vi "ACP Configure.vi"(0 "RFmx Handle In":refnum<k21>, 1 "Selector String":string, 5 "RFmx LTE ACP Configuration":T1={"Measurement Enabled"=TRUE, "Number of GSM Offsets"=0, "Number of UTRA Offsets"=2, "Number of EUTRA Offsets"=1, "Sweep Time Auto"=1, "Sweep Time Interval (s)"=0.001, "Averaging Enabled"=0, "Averaging Count"=10, "Averaging Type"=0, "RBW Auto"=1, "RBW (Hz)"=30000.0, "RBW Filter Type"=0} {"RBW Filter Type" items=["FFT Based", "Gaussian", "Flat"]; "RBW Auto" items=["False", "True"]; "Averaging Type" items=["False", "True"]; "Averaging Enabled" items=["False", "True"]; "Sweep Time Auto" items=["False", "True"]}, 11 "error in (no error)":errorcluster) -> (4 "RFmx Handle Out":refnum<k21>, 15 "error out":errorcluster)   [LabVIEW 2018, in "RFmxLTE.lvlib"]
uses:
  RFmxLTE.lvlib
  Typedefs/ACP Configuration.ctl
  <resource>/objmgr/RFmxLTE.rc
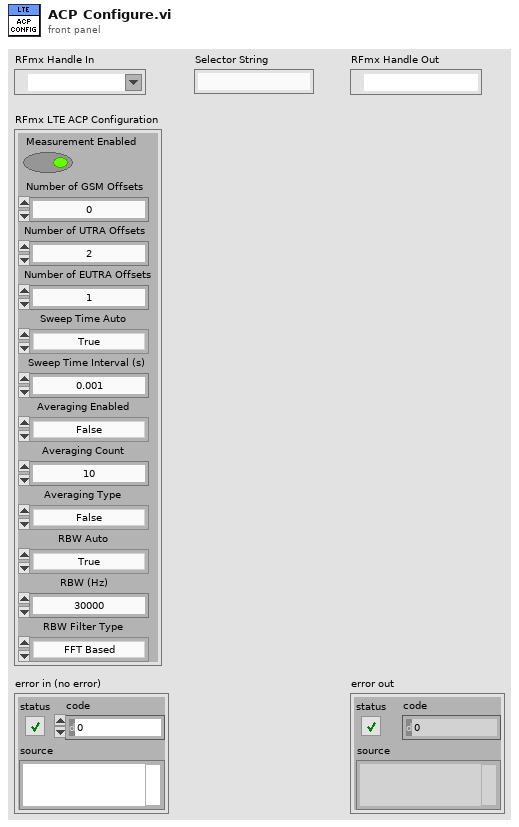
[diagram p1: front panel]
types:
  T1 = typedef "RFmxLTE.lvlib/ACP Configuration.ctl" = cluster{"Measurement Enabled":bool, "Number of GSM Offsets":i32, "Number of UTRA Offsets":i32, "Number of EUTRA Offsets":i32, "Sweep Time Auto":i32, "Sweep Time Interval (s)":dbl, "Averaging Enabled":i32, "Averaging Count":i32, "Averaging Type":i32, "RBW Auto":i32, "RBW (Hz)":dbl, "RBW Filter Type":i32}
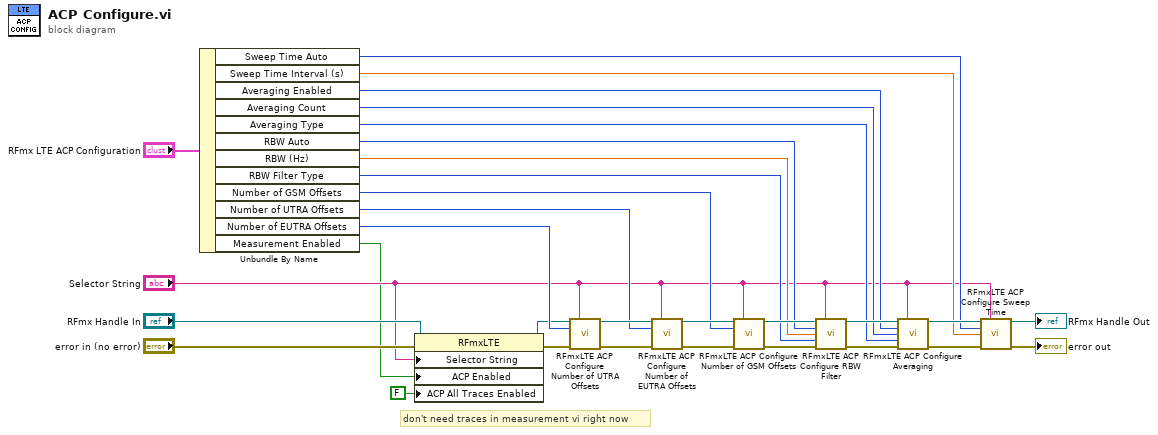
[diagram p0: block diagram]
diagram:
  # "don't need traces in measurement vi right now"
  n1 = Unbundle By Name("RFmx LTE ACP Configuration") -> ("Sweep Time Auto"=w18:i32, "Sweep Time Interval (s)"=w17:dbl, "Averaging Enabled"=w16:i32, "Averaging Count"=w15:i32, "Averaging Type"=w14:i32, "RBW Auto"=w13:i32, "RBW (Hz)"=w12:dbl, "RBW Filter Type"=w11:i32, "Number of GSM Offsets"=w10:i32, "Number of UTRA Offsets"=w9:i32, "Number of EUTRA Offsets"=w8:i32, "Measurement Enabled"=w2:bool)
  n2 = property class="RFmxLTE"(reference="RFmx Handle In", error in="error in (no error)", "Selector String"="Selector String", "ACP Enabled"=w2, "ACP All Traces Enabled"=FALSE) -> (reference out=w4:refnum<k21>, error out=w6:errorcluster)
  n3 = call <vilib>:"RFmxLTE ACP Configure Number of UTRA Offsets.vi"("Instrument Handle In"=w4, "Selector String"="Selector String", "Number of UTRA Offsets"=w8, "error in (no error)"=w6) -> ("Instrument Handle Out"=w31:refnum<k21>, "error out"=w30:errorcluster)  [unwired: 10 in]
  n4 = call <vilib>:"RFmxLTE ACP Configure Number of EUTRA Offsets.vi"("Instrument Handle In"=w31, "Selector String"="Selector String", "Number of EUTRA Offsets"=w9, "error in (no error)"=w30) -> ("Instrument Handle Out"=w29:refnum<k21>, "error out"=w28:errorcluster)  [unwired: 10 in]
  n5 = call <vilib>:"RFmxLTE ACP Configure Number of GSM Offsets.vi"("Instrument Handle In"=w29, "Selector String"="Selector String", "Number of GSM Offsets"=w10, "error in (no error)"=w28) -> ("Instrument Handle Out"=w27:refnum<k21>, "error out"=w26:errorcluster)  [unwired: 10 in]
  n6 = call <vilib>:"RFmxLTE ACP Configure RBW Filter.vi"("Instrument Handle In"=w27, "Selector String"="Selector String", "RBW Auto"=w13, "RBW (Hz)"=w12, "RBW Filter Type"=w11, "error in (no error)"=w26) -> ("Instrument Handle Out"=w25:refnum<k21>, "error out"=w24:errorcluster)  [unwired: 8 in]
  n7 = call <vilib>:"RFmxLTE ACP Configure Averaging.vi"("Instrument Handle In"=w25, "Selector String"="Selector String", "Averaging Enabled"=w16, "Averaging Count"=w15, "Averaging Type"=w14, "error in (no error)"=w24) -> ("Instrument Handle Out"=w23:refnum<k21>, "error out"=w22:errorcluster)  [unwired: 8 in]
  n8 = call <vilib>:"RFmxLTE ACP Configure Sweep Time.vi"("Instrument Handle In"=w23, "Selector String"="Selector String", "Sweep Time Auto"=w18, "Sweep Time Interval (s)"=w17, "error in (no error)"=w22) -> ("Instrument Handle Out"=→"RFmx Handle Out":refnum<k21>, "error out"=→"error out":errorcluster)  [unwired: 9 in]
